vi "Begin.vi"(8 "error in (no error)":errorcluster, 9 "Pneumatics control.lvlib:Solenoids.lvclass":refnum<class "Solenoids.lvclass">, 10 "Settings":variant, 11 "Pneumatics in":refnum<class "Pneumatics.lvclass">) -> (0 "error out":errorcluster, 3 "Pneumatics out":refnum<class "Pneumatics.lvclass">)   [LabVIEW 2018, in "Pneumatics control.lvlib" / "Pneumatics.lvclass"]
doc: "This VI instantiates the solenoids in the pnaumatic class, and sets both the channels and the PCM id based on the configuration input we receive."
uses:
  Pneumatics.lvclass
  Solenoids/Solenoids.lvclass
  TypeDefs/Solenoids.ctl
  Pneumatics.lvclass/Pneumatics.ctl
  df110fe4-3670-4473-9499-9f180371a8d4.vi
  <vilib>/Utility/error.llb/Trim Whitespace.vi
  <vilib>/Utility/error.llb/Error Cluster From Error Code.vi
  <vilib>/Rock Robotics/WPI/Utilities/WPI_GetSetVariantRefNum.vi
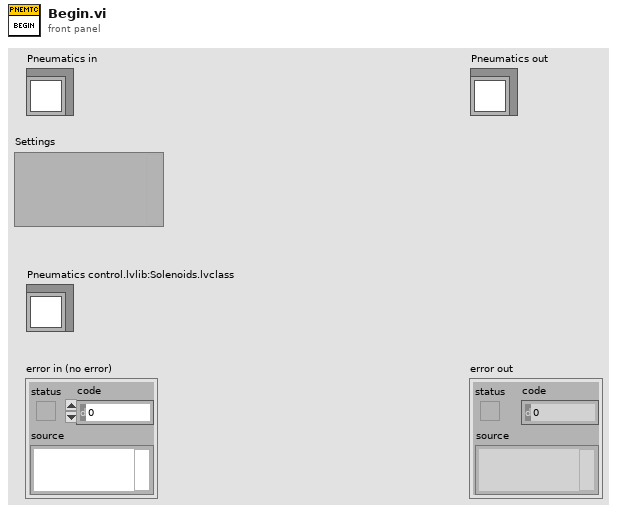
[diagram p1: front panel]
types:
  T1 = typedef "Pneumatics control.lvlib/Pneumatics.lvclass/Solenoids.ctl" = cluster{"DriveShift":refnum<class "Solenoids.lvclass">, "ArmLock":refnum<class "Solenoids.lvclass">, "HatchArm":refnum<class "Solenoids.lvclass">, "HatchGrabber":refnum<class "Solenoids.lvclass">}
  T2 = typedef "WPI_CompressorDevRef.ctl" = cluster{"DevStatus":errorcluster, "Pneumatics Control Module":u8}
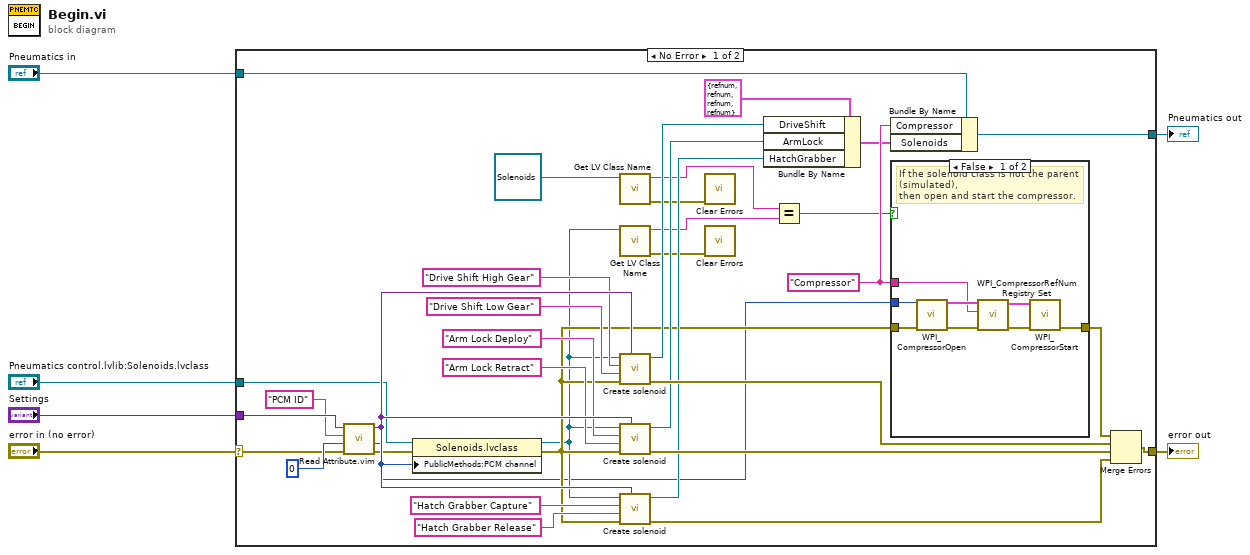
[diagram p0: block diagram]
diagram:
  n1 = case shown="No Error" "error in (no error)" {
    selector: "error in (no error)" -> [w34 w52]
    tunnel: [w30 w52] -> w5
    tunnel: [w40 w51] -> w3
    tunnel: "Pneumatics in" -> [w41 w51]
    tunnel: "Settings" -> [w37 _]
    tunnel: "Pneumatics control.lvlib:Solenoids.lvclass" -> [w9 _]
    frame No Error {
      w39 = "Compressor" ("refnum name")
      n2 = call "Read Attribute.vim"("error in"=w34, "default value (data type)"=u8 0, "name"="PCM ID", "variant in"=w37) -> ("error out"=w27:errorcluster, "value"=w7:u8, "variant out"=w28:variant)  [unwired: 4 in, 1 out]
      n3 = property class="Solenoids.lvclass"(reference=w9, error in=w27, "PublicMethods:PCM channel"=w7) -> (reference out=w8:refnum<class "Solenoids.lvclass">, error out=w10:errorcluster)
      n4 = call <vilib>:"Get LV Class Name.vi"("object"=refnum<class "Solenoids.lvclass"> refnum ("Pneumatics control.lvlib:Solenoids.lvclass")) -> ("error out"=w12:errorcluster, "class name"=w15:string)  [unwired: 9 in]
      n5 = call <vilib>:"Get LV Class Name.vi"("object"=w8) -> ("error out"=w11:errorcluster, "class name"=w14:string)  [unwired: 9 in]
      n6 = call "Create solenoid.vi"("Variant"=w28, "error in (no error)"=w10, "Reverse solenoid channel"="Drive Shift Low Gear", "Forward solenoid channel"="Drive Shift High Gear", "Solenoids in"=w8) -> ("error out"=w29:errorcluster, "Solenoids out"=w31:refnum<class "Solenoids.lvclass">)  [unwired: 5 in]
      n7 = call "Create solenoid.vi"("Variant"=w28, "error in (no error)"=w10, "Reverse solenoid channel"="Arm Lock Retract", "Forward solenoid channel"="Arm Lock Deploy", "Solenoids in"=w8) -> ("error out"=w25:errorcluster, "Solenoids out"=w23:refnum<class "Solenoids.lvclass">)  [unwired: 5 in]
      n8 = call "Create solenoid.vi"("Variant"=w28, "error in (no error)"=w10, "Reverse solenoid channel"="Hatch Grabber Release", "Forward solenoid channel"="Hatch Grabber Capture", "Solenoids in"=w8) -> ("error out"=w26:errorcluster, "Solenoids out"=w24:refnum<class "Solenoids.lvclass">)  [unwired: 5 in]
      n9 = call <vilib>:"Clear Errors.vi"("error in (no error)"=w12) -> ()  [unwired: 5 in, 2 out]
      n10 = call <vilib>:"Clear Errors.vi"("error in (no error)"=w11) -> ()  [unwired: 5 in, 2 out]
      n11 = Bundle By Name(cluster=T1 {"DriveShift"=refnum, "ArmLock"=refnum, "HatchArm"=refnum, "HatchGrabber"=refnum} ("Solenoids"), "DriveShift"=w31, "ArmLock"=w23, "HatchGrabber"=w24) -> (w32:T1)
      n12 = Equal?(x=w15, y=w14) -> (x = y?=w13:bool)
      n13 = Bundle By Name(cluster=w41, "Compressor"=w39, "Solenoids"=w32) -> (w40:refnum<class "Pneumatics.lvclass">)
      n14 = case shown="False" w13 {
        tunnel: w39 -> [w45 _]
        tunnel: [w44 w50] -> w38
        tunnel: w10 -> [w43 w50]
        tunnel: w7 -> [w42 _]
        frame False {
          # "If the solenoid class is not the parent (simulated),\nthen open and start the compressor."
          n15 = call <vilib>:"WPI_CompressorOpen.vi"("Pneumatics Control Module (0)"=w42, "error in (no error)"=w43) -> ("CompressorDevRef"=w49:T2, "error out"=w47:errorcluster)  [unwired: 12 in]
          n16 = call <vilib>:"WPI_CompressorRefNum Registry Set.vi"("error in (no error)"=w47, "refnum name"=w45, "CompressorDevRef"=w49) -> ("error out"=w46:errorcluster, "CompressorDevRef"=w48:T2)  [unwired: 7 in]
          n17 = call <vilib>:"WPI_CompressorStart.vi"("error in (no error)"=w46, "CompressorDevRef"=w48) -> ("error out"=w44:errorcluster)  [unwired: 8 in, 1 out]
        }
        frame True {
          # "If simulated, then do not open the compressor"
        }
      }
      n18 = Merge Errors(w38, w29, w25, w26) -> (w30:errorcluster)
    }
    frame Error {
    }
  }
  "error out" <- w5
  "Pneumatics out" <- w3
